vi "GUI Pump Station Indicator.vi"() -> ()   [LabVIEW 2019]
uses:
  TypeDef/GUI Pop Out.ctl
panel:
  in  "Pop-Out":T1
  out "DI 7":bool=TRUE caption="Низкий уровень\nавария"
  in  "State 2":string="Авария / Предупреждение / Ок" caption="State"
  out "Boolean Round":bool=TRUE
  in  "State":string="Отключенна"
  out "Vertical Fill Indicator":dbl(slide)=5.954198473282443 caption="Температура масла" scale=0.0..100.0
  out "Уровень  масла":dbl(slide)=37.72455089820359 scale=0.0..100.0
  in  "String":string="Гидростанция очистки и охлаждения"
  # "Насос перекачки в бак подачи"
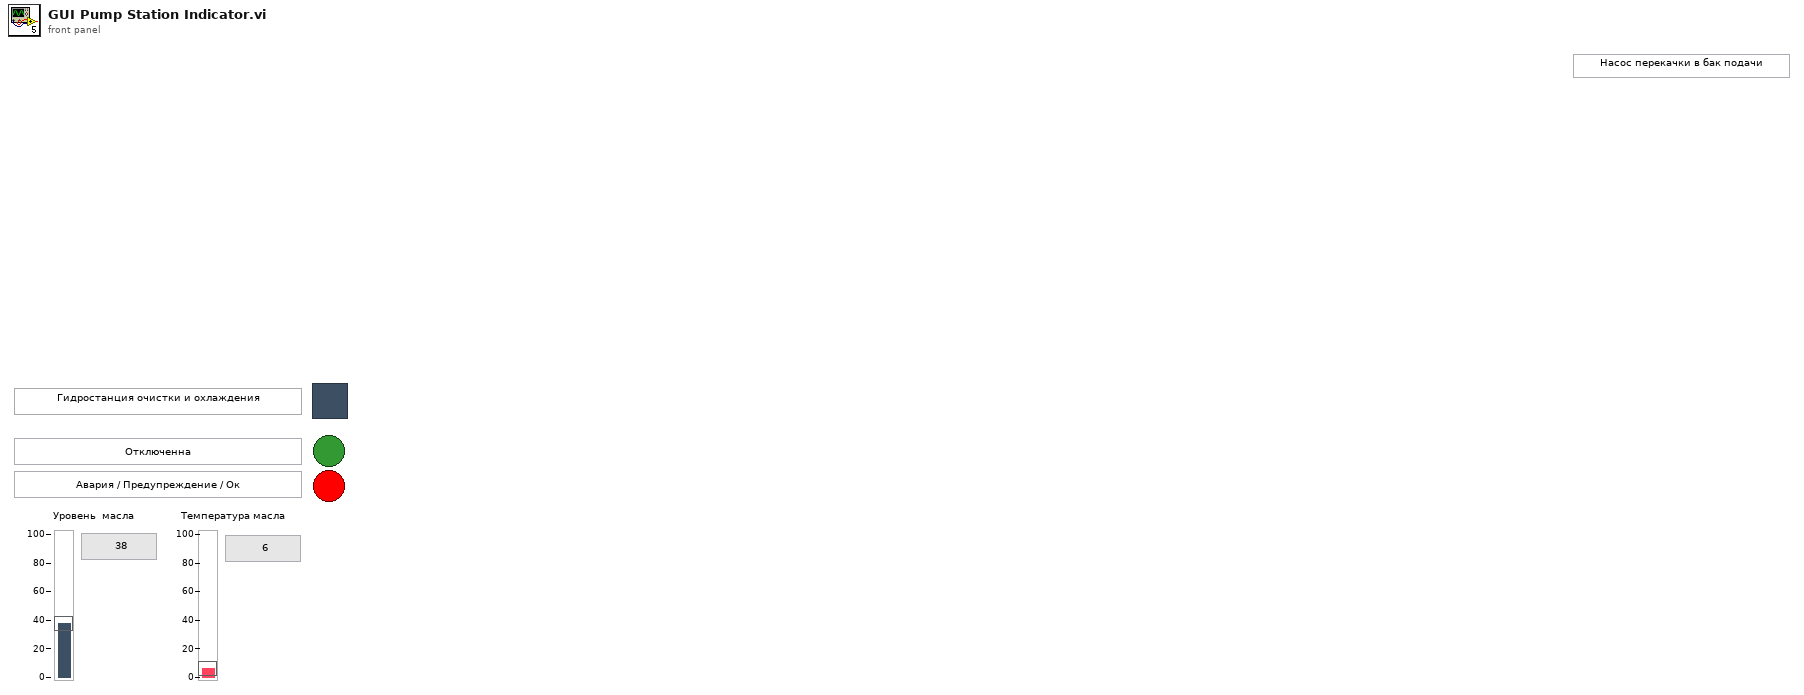
[diagram p1: front panel]
types:
  T1 = typedef "GUI Pop Out.ctl" = bool
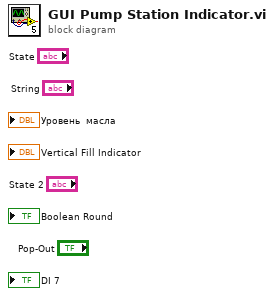
[diagram p0: block diagram]
diagram:
